vi "barcodeR92A.vi"(8 "主码":string, 10 "固定码":cluster{"start row":i32, "start column":i32}={"start row"=2, "start column"=1}) -> (2 "R92A二维码":string)   [LabVIEW 2018]
panel:
  out "结果字符串":string
  out "校验码":string
  out "校验码数组":string[](array[string])=["0", "1", "2", "3", "4", "5", "6", "7", "8", "9", "A", "B", "C", "D", "E", "F", "G", "H", "J", "K", "L", "M", "N", "P", "R", "S", "T", "U", "V", "W", "X", "Y", "Z"]
  out "月份字码对照月校验数组":string[](array[string])=["", "", "", "", "", "", "", "", "", "", "01", "02", "03", "04", "05", "06", "07", "08", "09", "10", "11", "12"]
  out "批次流水号码":string
  out "年月日":string
  out "年月日时分码":string
  out "日期/时间字符串":string
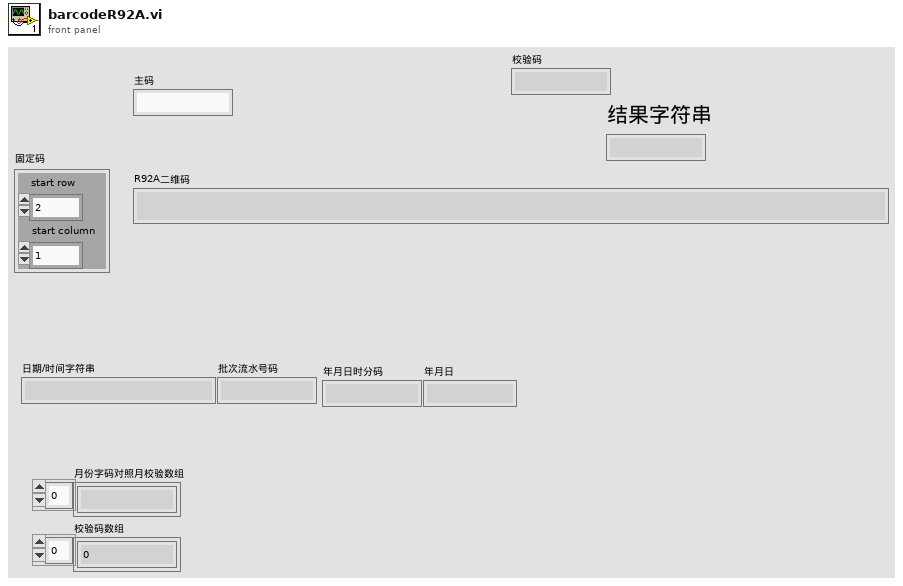
[diagram p1: front panel]
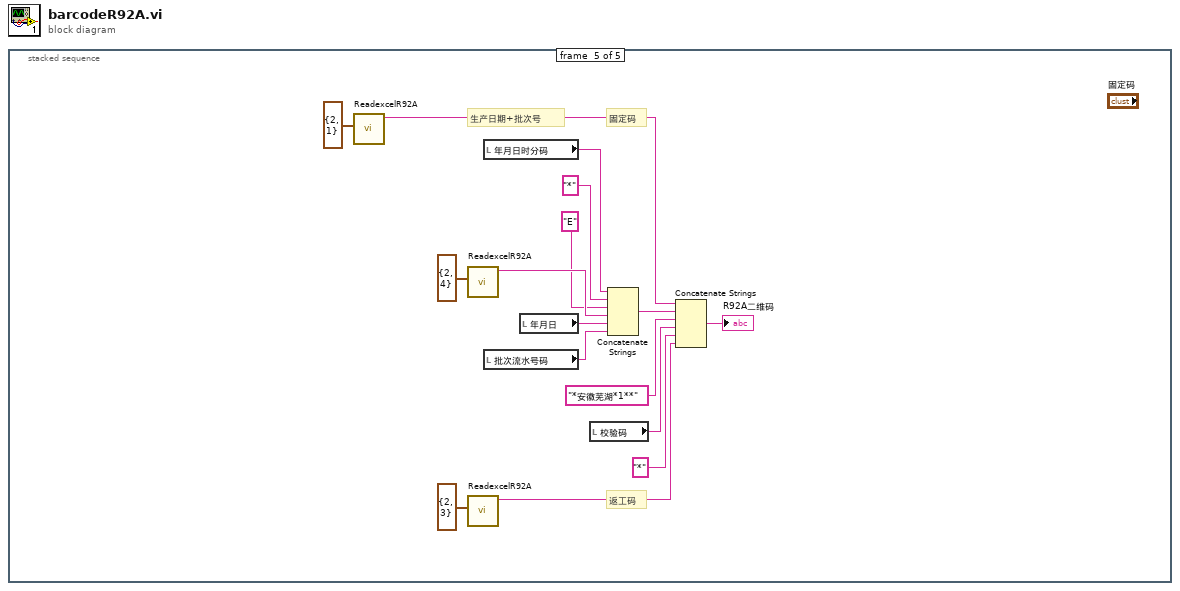
[diagram p0: block diagram]
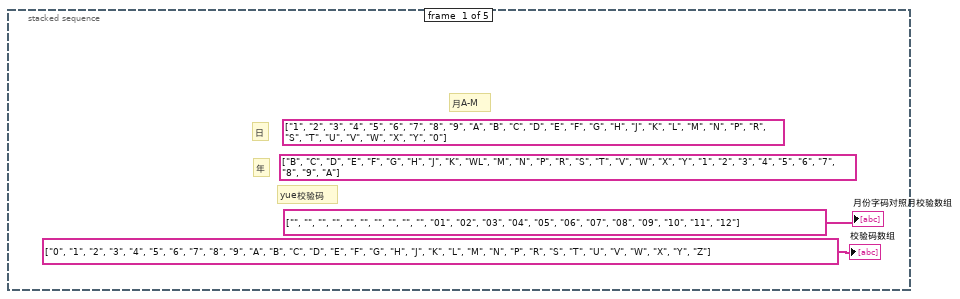
[diagram p2: hidden frame]
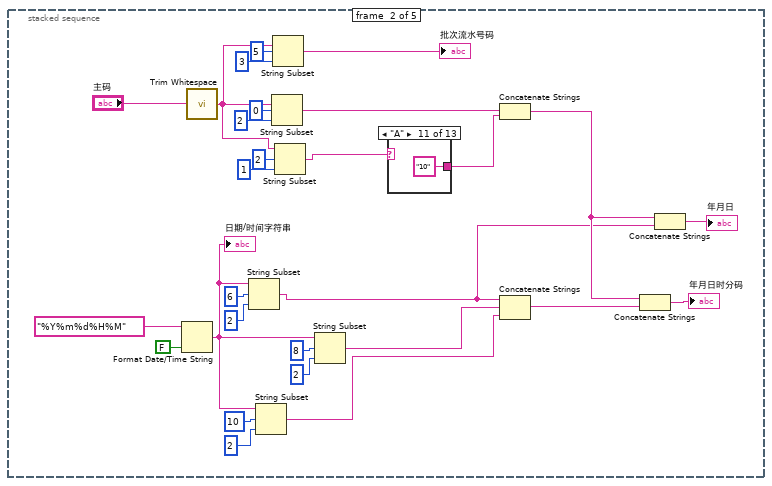
[diagram p3: hidden frame]
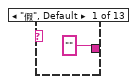
[diagram p4: hidden frame]
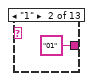
[diagram p5: hidden frame]
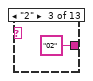
[diagram p6: hidden frame]
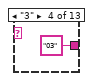
[diagram p7: hidden frame]
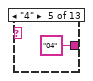
[diagram p8: hidden frame]
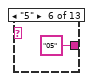
[diagram p9: hidden frame]
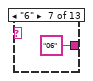
[diagram p10: hidden frame]
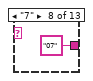
[diagram p11: hidden frame]
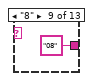
[diagram p12: hidden frame]
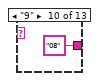
[diagram p13: hidden frame]
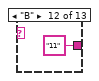
[diagram p14: hidden frame]
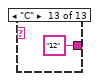
[diagram p15: hidden frame]
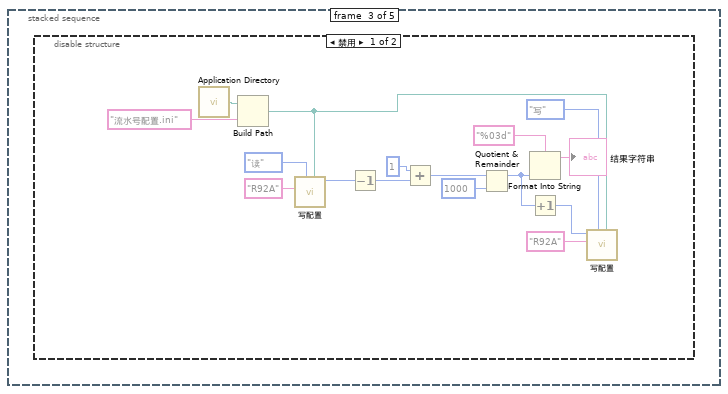
[diagram p16: hidden frame]
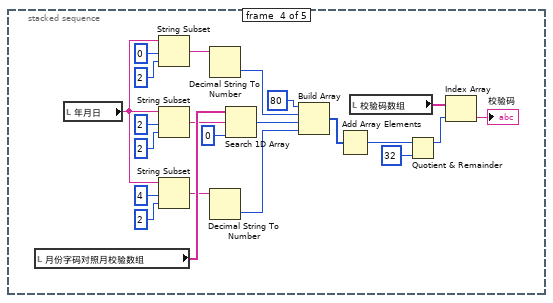
[diagram p18: hidden frame]
diagram:
  n1 = stacked-sequence {
    frame #0 {
      (unwired) string[] ["B", "C", "D", "E", "F", "G", "H", "J", "K", "WL", "M", "N", "P", "R", "S", "T", "V", "W", "X", "Y", "1", "2", "3", "4", "5", "6", "7", "8", "9", "A"]
      (unwired) string[] ["1", "2", "3", "4", "5", "6", "7", "8", "9", "A", "B", "C", "D", "E", "F", "G", "H", "J", "K", "L", "M", "N", "P", "R", "S", "T", "U", "V", "W", "X", "Y", "0"]
      # "月A-M"
      # "yue校验码"
      # "日"
      # "年"
      "月份字码对照月校验数组" <- string[] ["", "", "", "", "", "", "", "", "", "", "01", "02", "03", "04", "05", "06", "07", "08", "09", "10", "11", "12"]
      "校验码数组" <- string[] ["0", "1", "2", "3", "4", "5", "6", "7", "8", "9", "A", "B", "C", "D", "E", "F", "G", "H", "J", "K", "L", "M", "N", "P", "R", "S", "T", "U", "V", "W", "X", "Y", "Z"]
    }
    frame #1 {
      n2 = Format Date/Time String(time format string (%c)="%Y%m%d%H%M" ("时间格式字符串(%c)"), UTC format=FALSE ("UTC格式")) -> (date/time string=w30:string)  [unwired: 1 in]
      "日期/时间字符串" <- w30
      n3 = call <vilib>:"Trim Whitespace.vi"("string"="主码") -> ("trimmed string"=w6:string)  [unwired: 1 in]
      n4 = String Subset(string=w30, offset (0)=6 ("偏移量(0)"), length (rest)=2 ("长度（剩余）")) -> (substring=w9:string)
      n5 = String Subset(string=w30, offset (0)=10 ("偏移量(0)"), length (rest)=2 ("长度（剩余）")) -> (substring=w3:string)
      n6 = String Subset(string=w6, offset (0)=0 ("偏移量(0)"), length (rest)=2 ("长度（剩余）")) -> (substring=w16:string)
      n7 = String Subset(string=w6, offset (0)=5 ("偏移量(0)"), length (rest)=3 ("长度（剩余）")) -> (substring=→"批次流水号码":string)
      n8 = String Subset(string=w6, offset (0)=2 ("偏移量(0)"), length (rest)=1 ("长度（剩余）")) -> (substring=w17:string)
      n9 = String Subset(string=w30, offset (0)=8 ("偏移量(0)"), length (rest)=2 ("长度（剩余）")) -> (substring=w4:string)
      n10 = case shown="\"A\"" w17 {
        tunnel: ["" "01" "02" "03" "04" "05" "06" "07" "08" "08" "10" "11" "12"] -> w15
        frame "假", Default {
        }
        frame "1" {
        }
        frame "2" {
        }
        frame "3" {
        }
        frame "4" {
        }
        frame "5" {
        }
        frame "6" {
        }
        frame "7" {
        }
        frame "8" {
        }
        frame "9" {
        }
        frame "A" {
        }
        frame "B" {
        }
        frame "C" {
        }
      }
      n11 = Concatenate Strings(w16, w15) -> (w10:string)
      n12 = Concatenate Strings(w9, w4, w3) -> (w14:string)
      n13 = Concatenate Strings(w10, w14) -> (→"年月日时分码":string)
      n14 = Concatenate Strings(w10, w9) -> (→"年月日":string)
    }
    frame #2 {
      n15 = disable-structure shown="禁用" {
        frame Disabled {
          n16 = call <vilib>:"Application Directory.vi"() -> ("Application Directory"=w58:path)
          n17 = Build Path(base path=w58, name or relative path="流水号配置.ini" ("名称或相对路径")) -> (appended path=w57:path)
          n18 = call "写配置.vi"("配置文件路径"=w57, "枚举"=enum16{"写", "读"}."读", "section"="R92A") -> ("读取值"=w56:u32)  [unwired: 8 in]
          n19 = Decrement(x=w56) -> (x-1=w55:u32)
          n20 = Add(x=u32 1, y=w55) -> (x+y=w59:u32)
          n21 = Quotient & Remainder(x=w59, y=u32 1000) -> (x-y*floor(x/y)=w54:u32)  [unwired: 1 out]
          n22 = Format Into String(format string="%03d" ("格式字符串"), w54) -> (resulting string=→"结果字符串":string)  [unwired: 2 in, 1 out]
          n23 = Increment(x=w54) -> (x+1=w53:u32)
          n24 = call "写配置.vi"("配置文件路径"=w57, "枚举"=enum16{"写", "读"}."写", "section"="R92A", "写入值"=w53) -> ()  [unwired: 7 in, 1 out]
        }
        frame Enabled {
        }
      }
    }
    frame #3 {
      n25 = local read "月份字码对照月校验数组"() -> (w78:string[])
      n26 = local read "年月日"() -> (w77:string)
      n27 = String Subset(string=w77, offset (0)=0 ("偏移量(0)"), length (rest)=2 ("长度（剩余）")) -> (substring=w71:string)
      n28 = String Subset(string=w77, offset (0)=2 ("偏移量(0)"), length (rest)=2 ("长度（剩余）")) -> (substring=w72:string)
      n29 = String Subset(string=w77, offset (0)=4 ("偏移量(0)"), length (rest)=2 ("长度（剩余）")) -> (substring=w75:string)
      n30 = Decimal String To Number(string=w71) -> (number=w73:i32)  [unwired: 2 in, 1 out]
      n31 = Decimal String To Number(string=w75) -> (number=w76:i32)  [unwired: 2 in, 1 out]
      n32 = Search 1D Array(1D array=w78, element=w72, start index (0)=0 ("开始索引(0)")) -> (index of element=w74:i32)
      n33 = Build Array(80 ("元素"), w73, w74, w76) -> (w81:i32[])
      n34 = Add Array Elements(numeric array=w81) -> (sum=w69:i32)
      n35 = local read "校验码数组"() -> (w79:string[])
      n36 = Quotient & Remainder(x=w69, y=32) -> (x-y*floor(x/y)=w70:i32)  [unwired: 1 out]
      n37 = Index Array(array=w79, index=w70) -> (element=→"校验码":string)
    }
    frame #4 {
      # "返工码"
      # "生产日期+批次号"
      # "固定码"
      n38 = call "ReadexcelR92A.vi"("start (0, 0)"=cluster{"start row":i32, "start column":i32} {"start row"=2, "start column"=1}) -> ("Excel设置码"=w89:string)  [unwired: 10 in]
      n39 = call "ReadexcelR92A.vi"("start (0, 0)"=cluster{"start row":i32, "start column":i32} {"start row"=2, "start column"=4}) -> ("Excel设置码"=w91:string)  [unwired: 10 in]
      n40 = call "ReadexcelR92A.vi"("start (0, 0)"=cluster{"start row":i32, "start column":i32} {"start row"=2, "start column"=3}) -> ("Excel设置码"=w90:string)  [unwired: 10 in]
      n41 = local read "年月日时分码"() -> (w95:string)
      n42 = local read "批次流水号码"() -> (w93:string)
      n43 = local read "年月日"() -> (w94:string)
      n44 = local read "校验码"() -> (w92:string)
      n45 = Concatenate Strings(w95, "*" ("字符串"), "E" ("字符串"), w91, w94, w93) -> (w96:string)
      n46 = Concatenate Strings(w89, w96, "*安徽芜湖*1**" ("字符串"), w92, "*" ("字符串"), w90) -> (→"R92A二维码":string)
    }
  }
